vi "Delete Temp Folders.vi"(8 "error in":errorcluster, 10 "relative path of LVLIB folders":path[](array[path]), 11 "custom device path":path) -> (0 "error out":errorcluster, 3 "custom device path out":path)   [LabVIEW 2020, in "Template Tool.lvlib"]
uses:
  Template Tool.lvlib
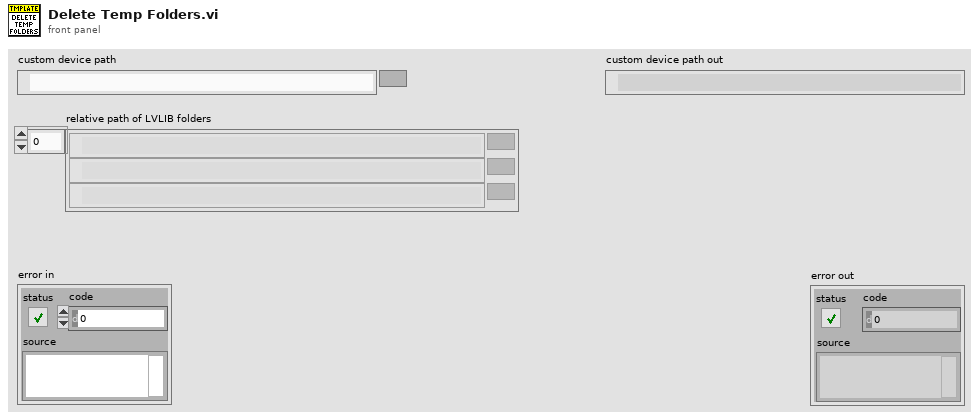
[diagram p1: front panel]
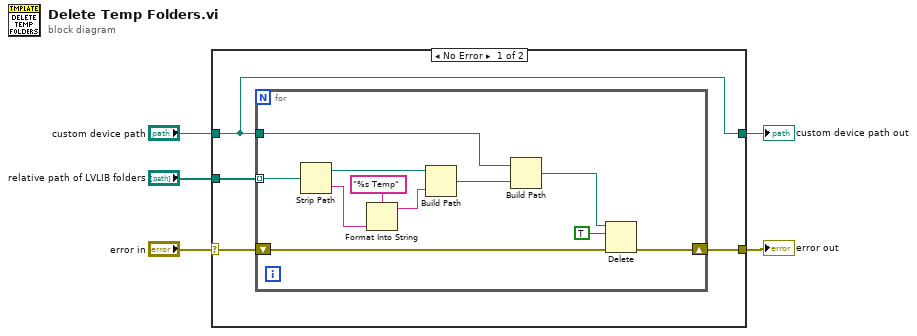
[diagram p0: block diagram]
diagram:
  n1 = case shown="No Error" "error in" {
    selector: "error in" -> [w9 w22]
    tunnel: "custom device path" -> [w7 w21]
    tunnel: [w8 w22] -> w4
    tunnel: [w7 w21] -> w3
    tunnel: "relative path of LVLIB folders" -> [w6 _]
    frame No Error {
      n2 = for {
        tunnel: w7 -> [w20]
        tunnel: w6 -> [w14] mode=indexing
        shift-right: [w17] -> w8
        shift-left: w9 -> [w18]
        n3 = Strip Path(path=w14) -> (stripped path=w13:path, name=w10:string)
        n4 = Format Into String(format string="%s Temp" ("string"), w10) -> (resulting string=w11:string)  [unwired: 2 in, 1 out]
        n5 = Build Path(base path=w13, name or relative path=w11) -> (appended path=w19:path)
        n6 = Build Path(base path=w20, name or relative path=w19) -> (appended path=w15:path)
        n7 = Delete(path (use dialog)=w15, entire hierarchy (F)=TRUE, error in=w18) -> (error out=w17:errorcluster)  [unwired: 2 in, 2 out]
      }
    }
    frame Error {
    }
  }
  "error out" <- w4
  "custom device path out" <- w3
